vi "Begin.vi"(8 "error in":errorcluster) -> (0 "error out":errorcluster)   [LabVIEW 2014]
doc: "Called before other user functions, this VI is expected to open initial I/O refnums, load in file data, and do all program initialization. Notice that the <B>error out</B> terminal is simply used for data flow. Wiring it to other structures or subVIs ensures that this VI runs first."
uses:
  <vilib>/Rock Robotics/WPI/DriverStation/WPI_DriverStationRobotMode2.ctl
  <vilib>/Rock Robotics/WPI/Joystick/WPI_JoystickDeviceEnum.ctl
  <vilib>/Rock Robotics/SystemInterfaces/AI/FPGA_AIGyroChannel.ctl
  <vilib>/Rock Robotics/SystemInterfaces/Typedef/FPGA_TypedefAnalogModuleForGyro.ctl
  <vilib>/Rock Robotics/SystemInterfaces/DIO/FPGA_DIOPWMChannel.ctl
  <vilib>/Rock Robotics/WPI/CAN/TalonSRX/WPI_CANTalonSRX_APIControlMode.ctl
  <vilib>/Rock Robotics/SystemInterfaces/DIO/FPGA_DIOChannel.ctl
  <vilib>/Rock Robotics/WPI/CAN/TalonSRX/WPI_CANTalonSRX_BrakeOverride.ctl
  Robot Global Data.vi
  <vilib>/Rock Robotics/Network Tables/SD Write String Array.vi
  <vilib>/Rock Robotics/WPI/MotorControl/WPI_MotorControlOpen Victor.vi
  <vilib>/Rock Robotics/WPI/MotorControl/WPI_MotorControlOpenCANTalonSRX.vi
  <vilib>/Rock Robotics/WPI/Counter/WPI_CounterDigitalInputToDigitalSource.vi
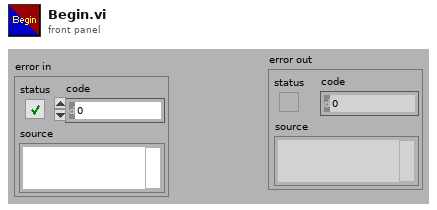
[diagram p1: front panel]
types:
  T1 = typedef "WPI_CANTalonSRX_BrakeOverride.ctl" = enum8{"No Override", "Override to Coast", "Override to Brake"}
  T2 = typedef "FPGA_DIOChannel.ctl" = enum8{"DIO 0", "DIO 1", "DIO 2", "DIO 3", "DIO 4", "DIO 5", "DIO 6", "DIO 7", "DIO 8", "DIO 9", "DIO MXP 0", "DIO MXP 1", "DIO MXP 2", "DIO MXP 3", "DIO MXP 4", "DIO MXP 5", "DIO MXP 6", "DIO MXP 7", "DIO MXP 8", "DIO MXP 9", "DIO MXP 10", "DIO MXP 11", "DIO MXP 12", "DIO MXP 13", "DIO MXP 14", "DIO MXP 15", "Invalid"}
  T3 = typedef "WPI_CANTalonSRX_APIControlMode.ctl" = enum8{"Percent VBus", "Speed", "Position", "Slave", "Unchanged / Invalid"}
  T4 = typedef "FPGA_DIOPWMChannel.ctl" = enum8{"PWM 0", "PWM 1", "PWM 2", "PWM 3", "PWM 4", "PWM 5", "PWM 6", "PWM 7", "PWM 8", "PWM 9", "PWM MXP 0", "PWM MXP 1", "PWM MXP 2", "PWM MXP 3", "PWM MXP 4", "PWM MXP 5", "PWM MXP 6", "PWM MXP 7", "PWM MXP 8", "PWM MXP 9", "Invalid"}
  T5 = typedef "FPGA_TypedefAnalogModuleForGyro.ctl" = enum16{"Controller 1"}
  T6 = typedef "FPGA_AIGyroChannel.ctl" = enum8{"AI 0", "AI 1", "Invalid"}
  T7 = typedef "WPI_JoystickDeviceEnum.ctl" = enum16{"USB 0", "USB 1", "USB 2", "USB 3", "USB 4", "USB 5"}
  T8 = typedef "WPI_DriverStationRobotMode2.ctl" = enum16{"Autonomous Disabled", "Autonomous Enabled", "Teleop Disabled", "Teleop Enabled", "Disconnected", "Finish", "Test Disabled", "Test Enabled", "Emergency Stopped"}
  T9 = typedef "WPI_DigitalInputDevRef.ctl" = cluster{"DevStatus":errorcluster, "DIO Channel":T2, "Controller":T10}
  T10 = typedef "FPGA_TypedefDigitalModule.ctl" = enum16{"Controller 1"}
  T11 = typedef "WPI_MotorControlDeviceRef.ctl" = cluster{"DeviceStatus":errorcluster, "Type":T12, "PWM":cluster{"Controller":T10, "PWM Channel":T4, "DeadBand":T13}, "CAN":cluster{"Device Number":u8, "Control Mode":T14, "Semaphore":T15, "Max Vout":dbl, "TalonSRX Control Mode":T3}, "Invert":bool, "TransformRef":T16, "InvTransformRef":T16}
  T12 = typedef "WPI_MotorControlType.ctl" = enum16{"PWM", "CAN", "CANTalonSRX"}
  T13 = typedef "WPI_PWMDeadband.ctl" = cluster{"Name":string, "maxPositivePwm":i32, "minPositivePwm":i32, "centerPwm":i32, "maxNegativePwm":i32, "minNegativePwm":i32, "angularRange":u16}
  T14 = typedef "WPI_CANJaguar_ControlMode.ctl" = enum8{"Percent VBus", "Current", "Speed", "Position", "Voltage"}
  T15 = typedef "Semaphore RefNum" = refnum<k1>
  T16 = typedef "WPI_PWMTransform_ConPane.ctl" = refnum<vi>
  T17 = typedef "WPI_GyroDevRef.ctl" = cluster{"DevStatus":errorcluster, "Analog Module":T18, "Analog Channel":T19, "Offset":dbl, "Gain (VoltsPerDegree/Second)":dbl}
  T18 = typedef "FPGA_TypedefAnalogModule.ctl" = enum16{"Controller 1"}
  T19 = typedef "FPGA_AIChannel.ctl" = enum8{"AI 0", "AI 1", "AI 2", "AI 3", "AI MXP 0", "AI MXP 1", "AI MXP 2", "AI MXP 3", "Invalid"}
  T20 = typedef "WPI_JoystickDevRef.ctl" = cluster{"Device":T7}
  T21 = typedef "FPGA_CounterEncoderSourceConvertionLVSourceType.ctl" = cluster{"DevStatus":errorcluster, "AnalogTriggerMode?":bool, "DigitalMode":cluster{"Controller":T10, "DIO Channel":T22}, "AnalogTriggerMode":cluster{"AnalogTriggerIndex":T23, "OutputType":T24}}
  T22 = typedef "FPGA_DIODigitalSourceChannel.ctl" = enum8{"DIO 0", "DIO 1", "DIO 2", "DIO 3", "DIO 4", "DIO 5", "DIO 6", "DIO 7", "DIO 8", "DIO 9", "DIO MXP 0", "DIO MXP 1", "DIO MXP 2", "DIO MXP 3", "DIO MXP 4", "DIO MXP 5", "DIO MXP 6", "DIO MXP 7", "DIO MXP 8", "DIO MXP 9", "DIO MXP 10", "DIO MXP 11", "DIO MXP 12", "DIO MXP 13", "DIO MXP 14", "DIO MXP 15", "Disabled"}
  T23 = typedef "FPGA_AnalogTriggerIndex.ctl" = enum8{"Trig 0", "Trig 1", "Trig 2", "Trig 3", "Trig 4", "Trig 5", "Trig 6", "Trig 7", "Invalid"}
  T24 = typedef "FPGA_AnalogTriggerOutType.ctl" = enum16{"InWindow", "TriggerState", "Rising", "Falling"}
  T25 = typedef "WPI_EncoderDevRef.ctl" = cluster{"DevStatus":errorcluster, "EncoderIndex":T26, "CounterIndex":T27, "DistancePerCount":dbl, "Decoding Type":T28}
  T26 = typedef "FPGA_EncoderIdx.ctl" = enum8{"Enc 0", "Enc 1", "Enc 2", "Enc 3", "Enc 4", "Enc 5", "Enc 6", "Enc 7", "Invalid"}
  T27 = typedef "FPGA_CounterCtrSystemIndex.ctl" = enum8{"Ctr 0", "Ctr 1", "Ctr 2", "Ctr 3", "Ctr 4", "Ctr 5", "Ctr 6", "Ctr 7", "Invalid"}
  T28 = typedef "WPI_EncoderType.ctl" = enum16{"1x", "2x", "4x"}
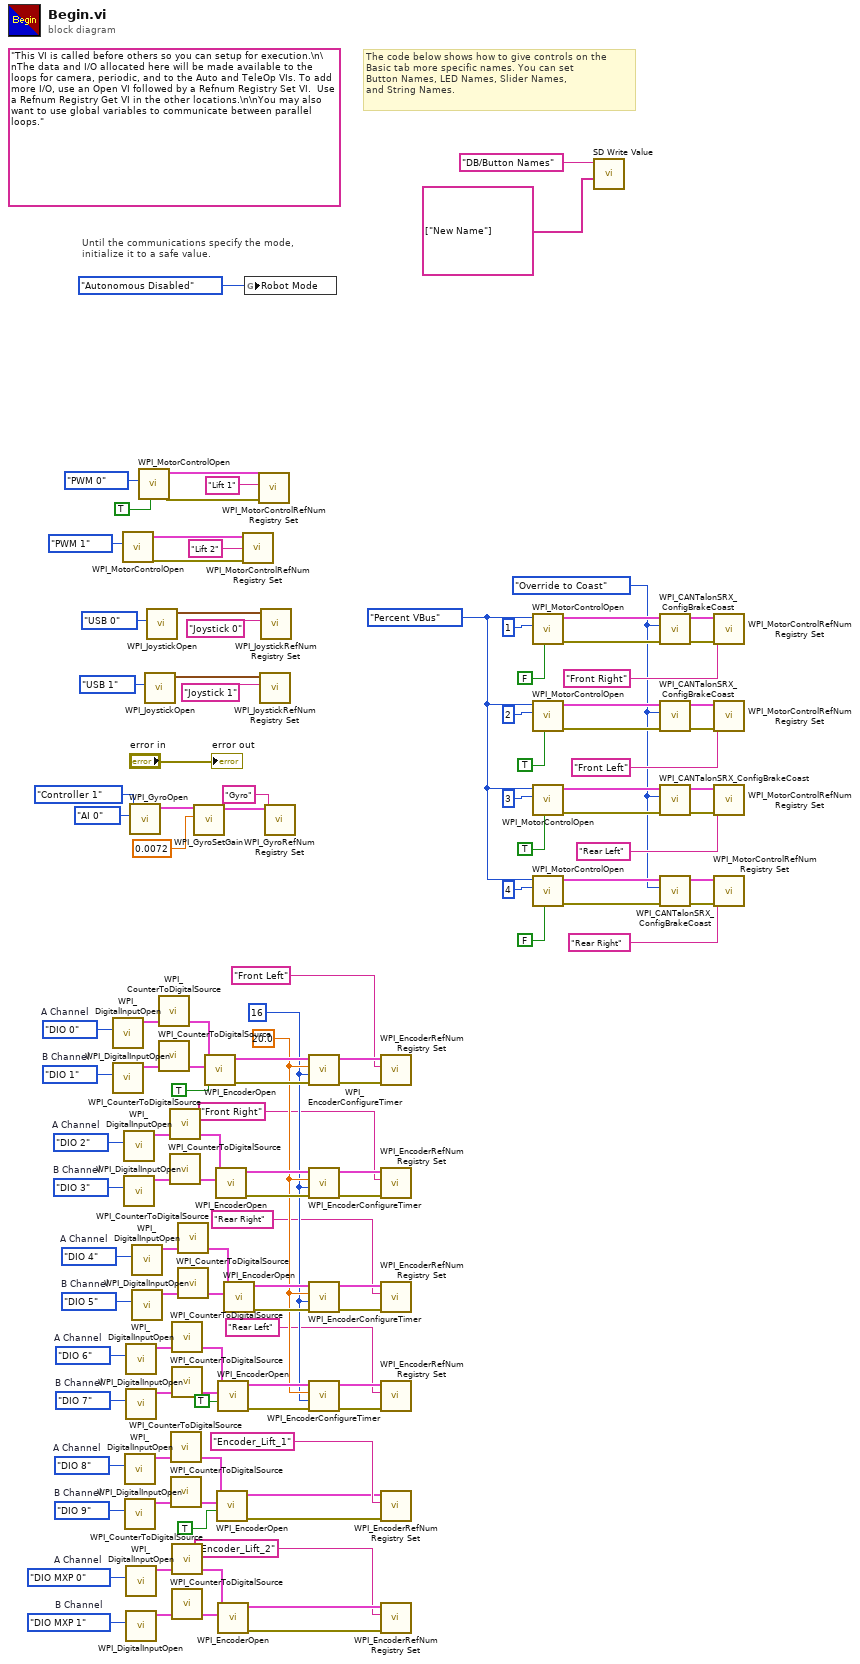
[diagram p0: block diagram]
diagram:
  w7 = u8 16 ("Number Samples to Average")
  w8 = 20.0 ("Minimum Rate")
  w29 = WPI_CANTalonSRX_BrakeOverride."Override to Coast" ("Brake / Coast Mode")
  w49 = FPGA_DIOChannel."DIO MXP 1"  # B Channel
  w50 = FPGA_DIOChannel."DIO MXP 0"  # A Channel
  w60 = FPGA_DIOChannel."DIO 9"  # B Channel
  w59 = FPGA_DIOChannel."DIO 8"  # A Channel
  w62 = FPGA_DIOChannel."DIO 7"  # B Channel
  w63 = FPGA_DIOChannel."DIO 6"  # A Channel
  w73 = FPGA_DIOChannel."DIO 5"  # B Channel
  w72 = FPGA_DIOChannel."DIO 4"  # A Channel
  w74 = FPGA_DIOChannel."DIO 3"  # B Channel
  w75 = FPGA_DIOChannel."DIO 2"  # A Channel
  w85 = FPGA_DIOChannel."DIO 1"  # B Channel
  w84 = FPGA_DIOChannel."DIO 0"  # A Channel
  w98 = WPI_CANTalonSRX_APIControlMode."Percent VBus" ("Control Mode")
  (unwired) "This VI is called before others so you can setup for execution.\n\nThe data and I/O allocated here will be made available to the loops for camera, periodic, and to the Auto and TeleOp VIs. To add more I/O, use an Open VI followed by a Refnum Registry Set VI.  Use a Refnum Registry Get VI in the other locations.\n\nYou may also want to use global variables to communicate between parallel loops."
  # "The code below shows how to give controls on the\nBasic tab more specific names. You can set\nButton Names, LED Names, Slider Names,\nand String Names."
  # "Until the communications specify the mode,\ninitialize it to a safe value."
  n1 = call <vilib>:"WPI_DigitalInputOpen.vi"("DIO Channel"=w84) -> ("DigitalInputDevRef"=w81:T9)  [unwired: 2 in, 8 out]
  n2 = call <vilib>:"WPI_DigitalInputOpen.vi"("DIO Channel"=w85) -> ("DigitalInputDevRef"=w82:T9)  [unwired: 2 in, 8 out]
  n3 = call-poly <vilib>:"WPI_MotorControlOpen.vi"("PWM Channel"=FPGA_DIOPWMChannel."PWM 1") -> ("error out"=w109:errorcluster, "MotorControlDeviceRef"=w108:T11)  [unwired: 9 in]
  n4 = call <vilib>:"WPI_DigitalInputOpen.vi"("DIO Channel"=w75) -> ("DigitalInputDevRef"=w78:T9)  [unwired: 2 in, 8 out]
  n5 = call <vilib>:"WPI_DigitalInputOpen.vi"("DIO Channel"=w74) -> ("DigitalInputDevRef"=w77:T9)  [unwired: 2 in, 8 out]
  n6 = call <vilib>:"WPI_DigitalInputOpen.vi"("DIO Channel"=w59) -> ("DigitalInputDevRef"=w56:T9)  [unwired: 2 in, 8 out]
  n7 = call <vilib>:"WPI_DigitalInputOpen.vi"("DIO Channel"=w60) -> ("DigitalInputDevRef"=w57:T9)  [unwired: 2 in, 8 out]
  n8 = call <vilib>:"WPI_DigitalInputOpen.vi"("DIO Channel"=w63) -> ("DigitalInputDevRef"=w66:T9)  [unwired: 2 in, 8 out]
  n9 = call <vilib>:"WPI_DigitalInputOpen.vi"("DIO Channel"=w62) -> ("DigitalInputDevRef"=w65:T9)  [unwired: 2 in, 8 out]
  n10 = call <vilib>:"WPI_DigitalInputOpen.vi"("DIO Channel"=w50) -> ("DigitalInputDevRef"=w53:T9)  [unwired: 2 in, 8 out]
  n11 = call <vilib>:"WPI_DigitalInputOpen.vi"("DIO Channel"=w49) -> ("DigitalInputDevRef"=w52:T9)  [unwired: 2 in, 8 out]
  n12 = call <vilib>:"WPI_GyroOpen.vi"("Analog Channel"=FPGA_AIGyroChannel."AI 0", "Controller"=FPGA_TypedefAnalogModuleForGyro."Controller 1") -> ("GyroDevRef"=w106:T17)  [unwired: 7 in, 2 out]
  n13 = call <vilib>:"WPI_DigitalInputOpen.vi"("DIO Channel"=w72) -> ("DigitalInputDevRef"=w69:T9)  [unwired: 2 in, 8 out]
  n14 = call <vilib>:"WPI_DigitalInputOpen.vi"("DIO Channel"=w73) -> ("DigitalInputDevRef"=w70:T9)  [unwired: 2 in, 8 out]
  n15 = call-poly <vilib>:"WPI_MotorControlOpen.vi"("Invert"=TRUE, "PWM Channel"=FPGA_DIOPWMChannel."PWM 0") -> ("error out"=w110:errorcluster, "MotorControlDeviceRef"=w112:T11)  [unwired: 8 in]
  n16 = call <vilib>:"WPI_JoystickOpen.vi"("JoystickDevice"=WPI_JoystickDeviceEnum."USB 1") -> ("JoystickDevRef"=w114:T20)  [unwired: 10 in]
  n17 = call <vilib>:"WPI_JoystickOpen.vi"("JoystickDevice"=WPI_JoystickDeviceEnum."USB 0") -> ("JoystickDevRef"=w120:T20)  [unwired: 10 in]
  n18 = call-poly <vilib>:"WPI_CounterToDigitalSource.vi"("DigitalInputDevRef"=w81) -> ("Digital Source"=w80:T21)  [unwired: 6 out]
  n19 = call-poly <vilib>:"WPI_CounterToDigitalSource.vi"("DigitalInputDevRef"=w82) -> ("Digital Source"=w83:T21)  [unwired: 6 out]
  n20 = call-poly <vilib>:"WPI_CounterToDigitalSource.vi"("DigitalInputDevRef"=w78) -> ("Digital Source"=w79:T21)  [unwired: 6 out]
  n21 = call-poly <vilib>:"WPI_CounterToDigitalSource.vi"("DigitalInputDevRef"=w77) -> ("Digital Source"=w76:T21)  [unwired: 6 out]
  n22 = call-poly <vilib>:"WPI_CounterToDigitalSource.vi"("DigitalInputDevRef"=w56) -> ("Digital Source"=w55:T21)  [unwired: 6 out]
  n23 = call-poly <vilib>:"WPI_CounterToDigitalSource.vi"("DigitalInputDevRef"=w57) -> ("Digital Source"=w58:T21)  [unwired: 6 out]
  n24 = call-poly <vilib>:"WPI_CounterToDigitalSource.vi"("DigitalInputDevRef"=w66) -> ("Digital Source"=w67:T21)  [unwired: 6 out]
  n25 = call-poly <vilib>:"WPI_CounterToDigitalSource.vi"("DigitalInputDevRef"=w65) -> ("Digital Source"=w64:T21)  [unwired: 6 out]
  n26 = call-poly <vilib>:"WPI_CounterToDigitalSource.vi"("DigitalInputDevRef"=w53) -> ("Digital Source"=w54:T21)  [unwired: 6 out]
  n27 = call-poly <vilib>:"WPI_CounterToDigitalSource.vi"("DigitalInputDevRef"=w52) -> ("Digital Source"=w51:T21)  [unwired: 6 out]
  n28 = call-poly <vilib>:"WPI_CounterToDigitalSource.vi"("DigitalInputDevRef"=w69) -> ("Digital Source"=w68:T21)  [unwired: 6 out]
  n29 = call-poly <vilib>:"WPI_CounterToDigitalSource.vi"("DigitalInputDevRef"=w70) -> ("Digital Source"=w71:T21)  [unwired: 6 out]
  n30 = call <vilib>:"WPI_GyroSetGain.vi"("Gain (VoltsPerDegree/Second)"=0.0072, "GyroDevRef"=w106) -> ("GyroDevRef"=w103:T17)  [unwired: 8 in, 1 out]
  n31 = call <vilib>:"WPI_EncoderOpen.vi"("Invert Direction (False)"=TRUE, "BSource"=w83, "ASource"=w80) -> ("error out"=w21:errorcluster, "EncoderDevRef"=w22:T25)  [unwired: 5 in, 2 out]
  n32 = call <vilib>:"WPI_EncoderOpen.vi"("BSource"=w76, "ASource"=w79) -> ("error out"=w18:errorcluster, "EncoderDevRef"=w20:T25)  [unwired: 6 in, 2 out]
  n33 = call <vilib>:"WPI_EncoderOpen.vi"("Invert Direction (False)"=TRUE, "BSource"=w58, "ASource"=w55) -> ("error out"=w25:errorcluster, "EncoderDevRef"=w26:T25)  [unwired: 5 in, 2 out]
  n34 = call <vilib>:"WPI_EncoderOpen.vi"("Invert Direction (False)"=TRUE, "BSource"=w64, "ASource"=w67) -> ("error out"=w10:errorcluster, "EncoderDevRef"=w12:T25)  [unwired: 5 in, 2 out]
  n35 = call <vilib>:"WPI_EncoderOpen.vi"("BSource"=w51, "ASource"=w54) -> ("error out"=w48:errorcluster, "EncoderDevRef"=w47:T25)  [unwired: 6 in, 2 out]
  n36 = call <vilib>:"WPI_EncoderOpen.vi"("BSource"=w71, "ASource"=w68) -> ("error out"=w15:errorcluster, "EncoderDevRef"=w16:T25)  [unwired: 6 in, 2 out]
  n37 = call <vilib>:"WPI_MotorControlRefNum Registry Set.vi"("error in (no error)"=w109, "refnum name"="Lift 2", "MotorControlDevRef"=w108) -> ()  [unwired: 7 in, 2 out]
  n38 = global write "Robot Global Data.vi" "Robot Mode"(WPI_DriverStationRobotMode2."Autonomous Disabled" ("Robot Mode")) -> ()
  n39 = call <vilib>:"WPI_MotorControlRefNum Registry Set.vi"("error in (no error)"=w110, "refnum name"="Lift 1", "MotorControlDevRef"=w112) -> ()  [unwired: 7 in, 2 out]
  n40 = call <vilib>:"WPI_JoystickRefNum Registry Set.vi"("refnum name"="Joystick 1", "JoystickDevRef"=w114) -> ()  [unwired: 8 in, 2 out]
  n41 = call <vilib>:"WPI_JoystickRefNum Registry Set.vi"("refnum name"="Joystick 0", "JoystickDevRef"=w120) -> ()  [unwired: 8 in, 2 out]
  n42 = call <vilib>:"WPI_GyroRefNum Registry Set.vi"("refnum name"="Gyro", "GyroDevRef"=w103) -> ()  [unwired: 8 in, 2 out]
  n43 = call <vilib>:"WPI_EncoderConfigureTimer.vi"("error in (no error)"=w21, "Number Samples to Average"=w7, "Minimum Rate"=w8, "EncoderDevRef"=w22) -> ("error out"=w23:errorcluster, "EncoderDevRef"=w24:T25)  [unwired: 6 in]
  n44 = call <vilib>:"WPI_EncoderConfigureTimer.vi"("error in (no error)"=w18, "Number Samples to Average"=w7, "Minimum Rate"=w8, "EncoderDevRef"=w20) -> ("error out"=w17:errorcluster, "EncoderDevRef"=w19:T25)  [unwired: 6 in]
  n45 = call <vilib>:"WPI_EncoderConfigureTimer.vi"("error in (no error)"=w15, "Number Samples to Average"=w7, "Minimum Rate"=w8, "EncoderDevRef"=w16) -> ("error out"=w13:errorcluster, "EncoderDevRef"=w14:T25)  [unwired: 6 in]
  n46 = call <vilib>:"WPI_EncoderConfigureTimer.vi"("error in (no error)"=w10, "Number Samples to Average"=w7, "Minimum Rate"=w8, "EncoderDevRef"=w12) -> ("error out"=w9:errorcluster, "EncoderDevRef"=w11:T25)  [unwired: 6 in]
  n47 = call <vilib>:"WPI_EncoderRefNum Registry Set.vi"("error in (no error)"=w23, "refnum name"="Front Left", "EncoderDevRef"=w24) -> ()  [unwired: 7 in, 2 out]
  n48 = call <vilib>:"WPI_EncoderRefNum Registry Set.vi"("error in (no error)"=w17, "refnum name"="Front Right", "EncoderDevRef"=w19) -> ()  [unwired: 7 in, 2 out]
  n49 = call <vilib>:"WPI_EncoderRefNum Registry Set.vi"("error in (no error)"=w13, "refnum name"="Rear Right", "EncoderDevRef"=w14) -> ()  [unwired: 7 in, 2 out]
  n50 = call <vilib>:"WPI_EncoderRefNum Registry Set.vi"("error in (no error)"=w9, "refnum name"="Rear Left", "EncoderDevRef"=w11) -> ()  [unwired: 7 in, 2 out]
  n51 = call <vilib>:"WPI_EncoderRefNum Registry Set.vi"("error in (no error)"=w25, "refnum name"="Encoder_Lift_1", "EncoderDevRef"=w26) -> ()  [unwired: 7 in, 2 out]
  n52 = call <vilib>:"WPI_EncoderRefNum Registry Set.vi"("error in (no error)"=w48, "refnum name"="Encoder_Lift_2", "EncoderDevRef"=w47) -> ()  [unwired: 7 in, 2 out]
  n53 = call-poly <vilib>:"WPI_MotorControlOpen.vi"("Invert"=FALSE, "Device Number"=u8 1, "Control Mode"=w98) -> ("error out"=w44:errorcluster, "MotorControlDeviceRef"=w45:T11)  [unwired: 7 in]
  n54 = call-poly <vilib>:"WPI_MotorControlOpen.vi"("Invert"=TRUE, "Device Number"=u8 2, "Control Mode"=w98) -> ("error out"=w38:errorcluster, "MotorControlDeviceRef"=w39:T11)  [unwired: 7 in]
  n55 = call-poly <vilib>:"WPI_MotorControlOpen.vi"("Invert"=TRUE, "Device Number"=u8 3, "Control Mode"=w98) -> ("error out"=w32:errorcluster, "MotorControlDeviceRef"=w33:T11)  [unwired: 7 in]
  n56 = call-poly <vilib>:"WPI_MotorControlOpen.vi"("Invert"=FALSE, "Device Number"=u8 4, "Control Mode"=w98) -> ("error out"=w37:errorcluster, "MotorControlDeviceRef"=w36:T11)  [unwired: 7 in]
  n57 = call-poly <vilib>:"SD Write Value.vi"("String Array"=string[] ["New Name"], "Name"="DB/Button Names") -> ()  [unwired: 8 in, 2 out]
  n58 = call <vilib>:"WPI_CANTalonSRX_ConfigBrakeCoast.vi"("error in (no error)"=w44, "Brake / Coast Mode"=w29, "CAN Talon SRX Ref"=w45) -> ("error out"=w43:errorcluster, "CAN Talon SRX Ref Out"=w42:T11)  [unwired: 7 in]
  n59 = call <vilib>:"WPI_CANTalonSRX_ConfigBrakeCoast.vi"("error in (no error)"=w38, "Brake / Coast Mode"=w29, "CAN Talon SRX Ref"=w39) -> ("error out"=w41:errorcluster, "CAN Talon SRX Ref Out"=w40:T11)  [unwired: 7 in]
  n60 = call <vilib>:"WPI_CANTalonSRX_ConfigBrakeCoast.vi"("error in (no error)"=w32, "Brake / Coast Mode"=w29, "CAN Talon SRX Ref"=w33) -> ("error out"=w31:errorcluster, "CAN Talon SRX Ref Out"=w30:T11)  [unwired: 7 in]
  n61 = call <vilib>:"WPI_CANTalonSRX_ConfigBrakeCoast.vi"("error in (no error)"=w37, "Brake / Coast Mode"=w29, "CAN Talon SRX Ref"=w36) -> ("error out"=w34:errorcluster, "CAN Talon SRX Ref Out"=w35:T11)  [unwired: 7 in]
  n62 = call <vilib>:"WPI_MotorControlRefNum Registry Set.vi"("error in (no error)"=w43, "refnum name"="Front Right", "MotorControlDevRef"=w42) -> ()  [unwired: 7 in, 2 out]
  n63 = call <vilib>:"WPI_MotorControlRefNum Registry Set.vi"("error in (no error)"=w41, "refnum name"="Front Left", "MotorControlDevRef"=w40) -> ()  [unwired: 7 in, 2 out]
  n64 = call <vilib>:"WPI_MotorControlRefNum Registry Set.vi"("error in (no error)"=w31, "refnum name"="Rear Left", "MotorControlDevRef"=w30) -> ()  [unwired: 7 in, 2 out]
  n65 = call <vilib>:"WPI_MotorControlRefNum Registry Set.vi"("error in (no error)"=w34, "refnum name"="Rear Right", "MotorControlDevRef"=w35) -> ()  [unwired: 7 in, 2 out]
  "error out" <- "error in"
